vi "main.vi"() -> ()   [LabVIEW 2016]
uses:
  AlCS/Subsystems.ctl
  ts_labview_tcp/TCPClient/TCPClient.lvclass
  C:/Users/aanania/Documents/ts_alignmentsystemclient/ts_labview_tcp/TCPCommunicator/TCPCommunicator.lvclass
  ts_labview_tcp/TCPComEvents/TCPComEvents.lvclass
  ts_labview_tcp/TCPSettings/TCPSettings.lvclass
  AlCS/AlCS.lvclass
  ts_labview_tcp/tcpTypedefs/TCPSettings.ctl
  View/View.lvclass
  ts_labview_tcp/TCPComEvents/TCPComEvents.lvclass/TCPComEvents.ctl
  ts_labview_tcp/TCPCommunicator/TCPCommunicator.lvclass/TCPCommunicator.ctl
  AlCS/AlCS.lvclass/AlCS.ctl
  Parser/CommandCreator.lvclass
  ts_labview_tcp/TCPCommunicator/TCPCommunicator.lvclass
panel:
  out "connectedClicked":bool
  in  "stop":bool
  in  "SubsystemsPosition":T1
  in  "QueryPosition":bool
  in  "QueryLaserStatus":bool
  in  "PowerLaserOff":bool
  in  "ClearError":bool
  in  "QueryStatus":bool
  in  "execMP":bool
  in  "SubsystemsMP":T1
  out "String":string
  out "Connected":bool
  in  "Disconnect":bool
  in  "Connect":bool
  in  "timeout (ms)":i32=1500
  in  "port":u16=50000
  in  "IP":string="localhost"
  # "TCP Settings"
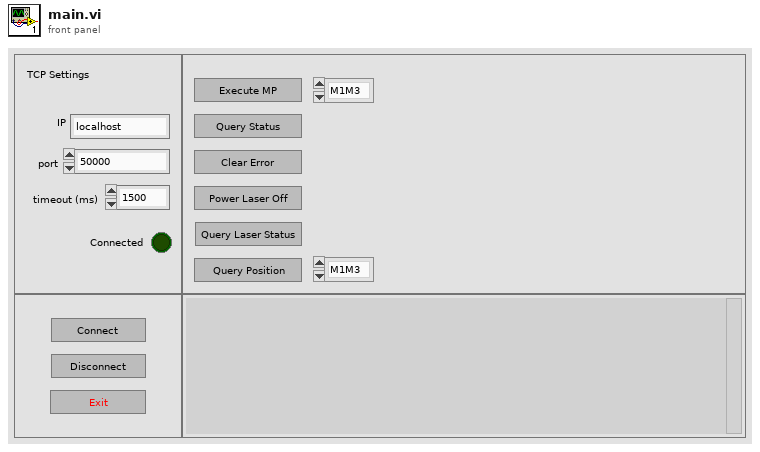
[diagram p1: front panel]
types:
  T1 = typedef "Subsystems.ctl" = enum16{"M1M3", "Camera", "M2"}
  T2 = typedef "TCPSettings.ctl" = cluster{"IP":string, "port_low":u16, "port_up":u16, "connection_timeout ":i32, "reading_timeout":i32, "writing_timeout":i32}
  T3 = cluster{"Subsystem":T1, "x":dbl, "y":dbl, "z":dbl, "rx":dbl, "ry":dbl, "rz":dbl}
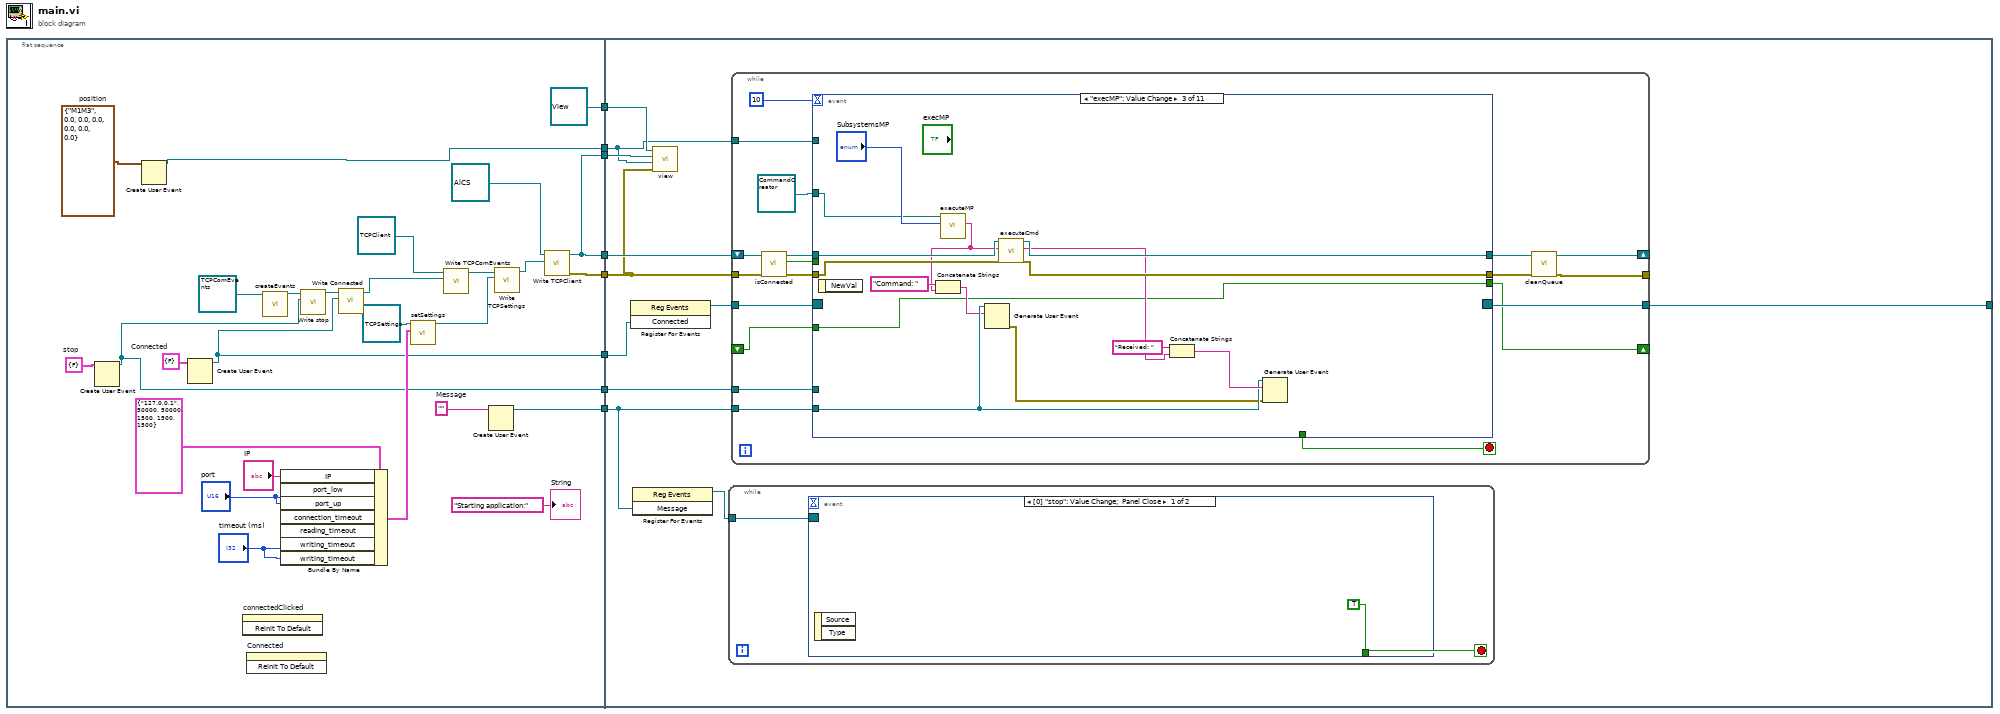
[diagram p0: block diagram]
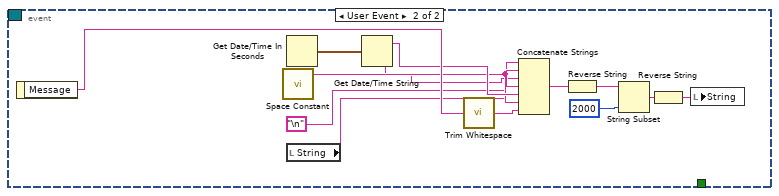
[diagram p2: hidden frame]
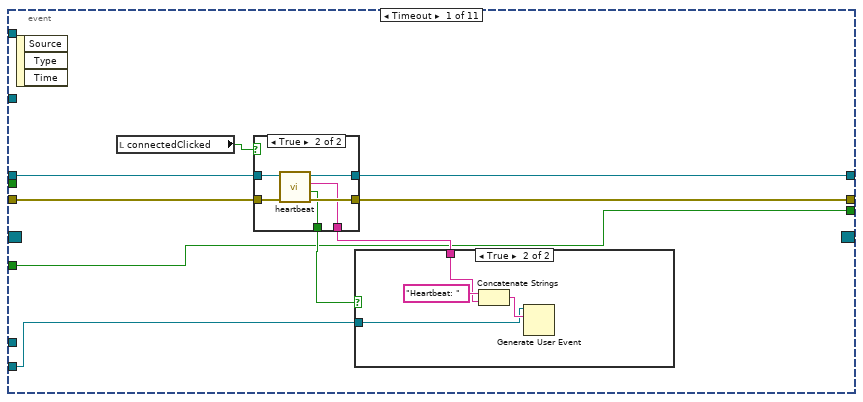
[diagram p3: hidden frame]
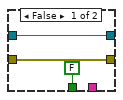
[diagram p5: hidden frame]
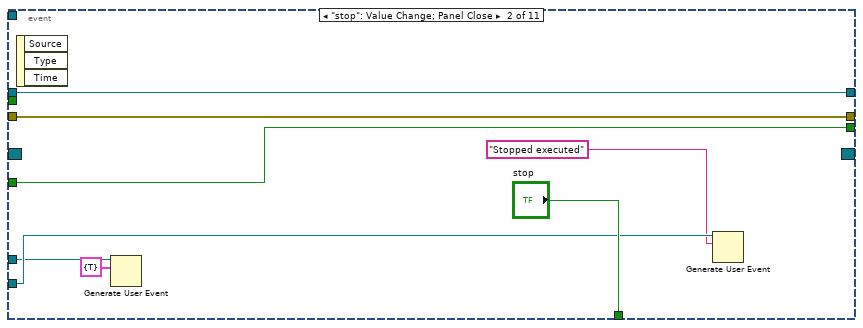
[diagram p6: hidden frame]
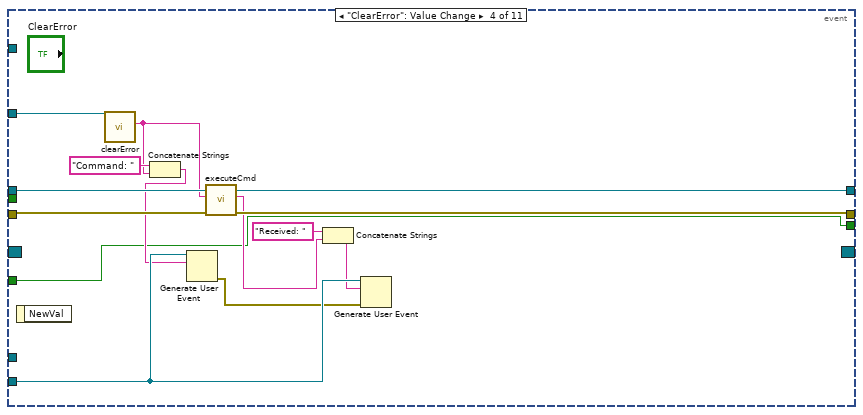
[diagram p7: hidden frame]
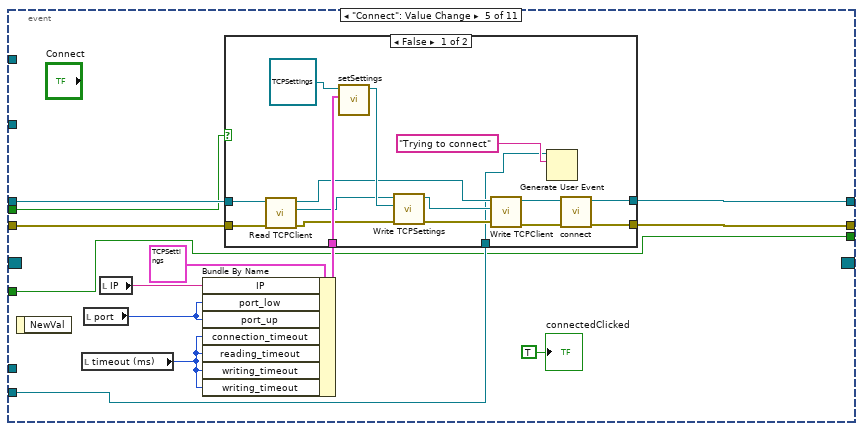
[diagram p8: hidden frame]
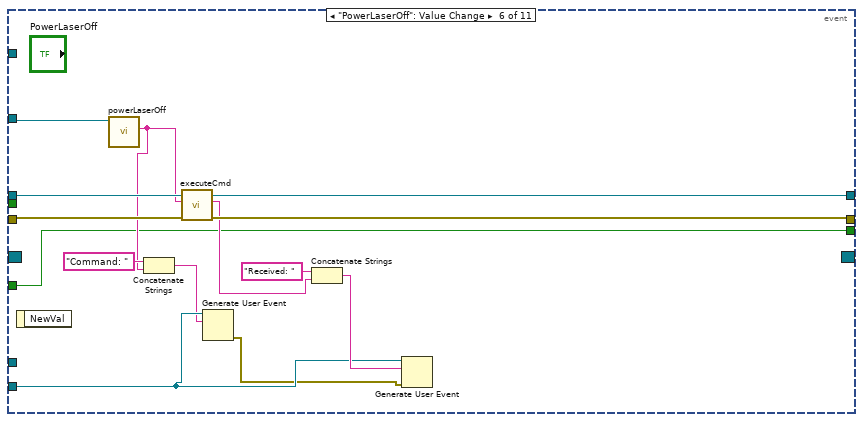
[diagram p10: hidden frame]
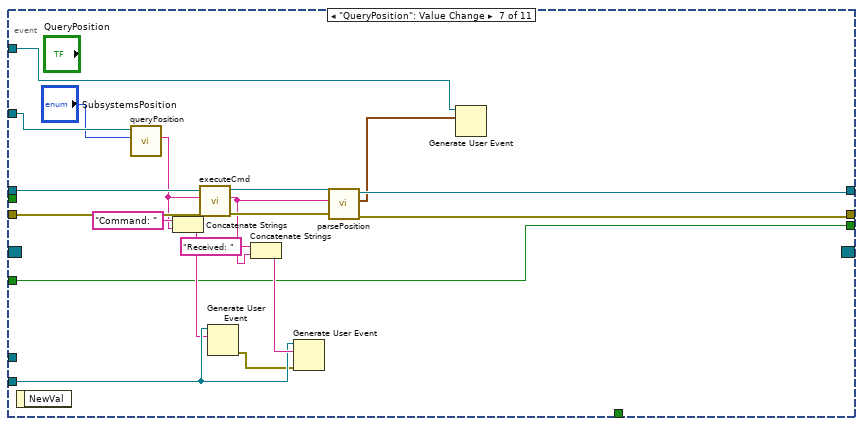
[diagram p11: hidden frame]
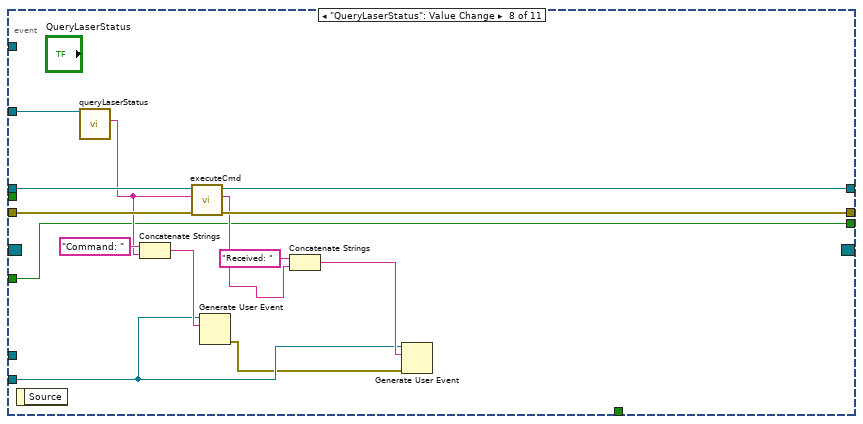
[diagram p12: hidden frame]
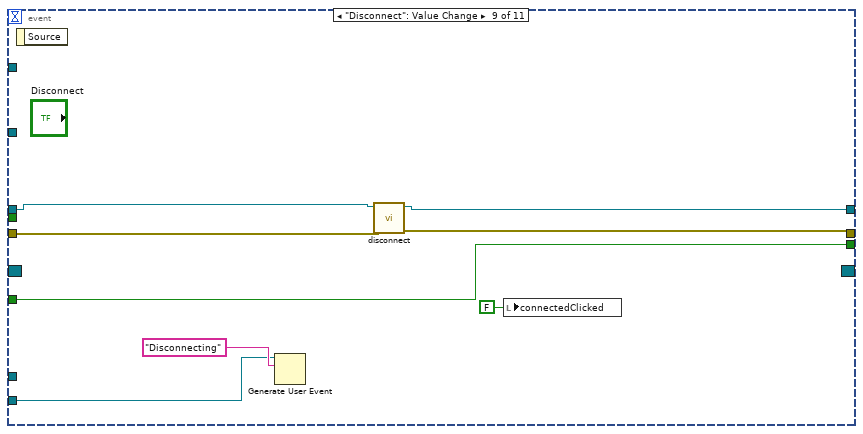
[diagram p13: hidden frame]
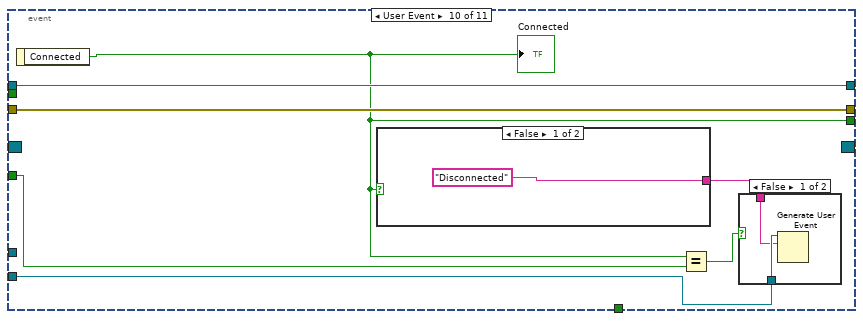
[diagram p14: hidden frame]
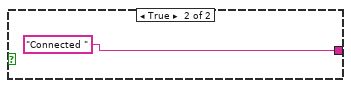
[diagram p16: hidden frame]
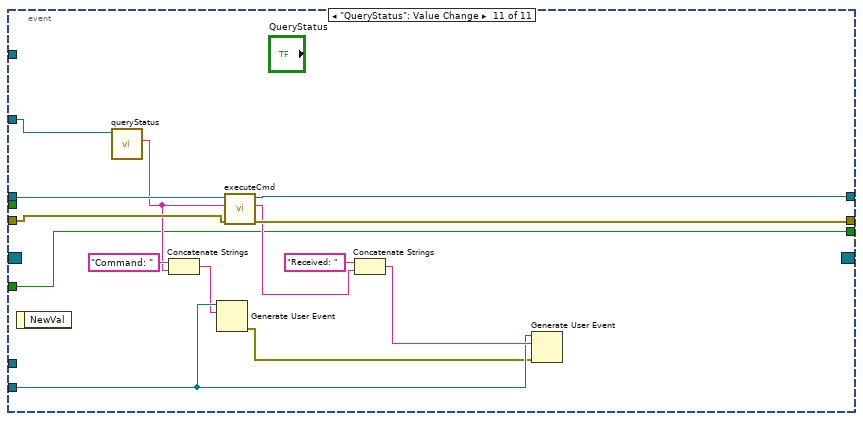
[diagram p17: hidden frame]
diagram:
  n1 = flat-sequence {
    tunnel: [w10] -> w8
    tunnel: [w19] -> w7
    tunnel: [w17] -> w6
    tunnel: [w16] -> w5
    tunnel: [w10] -> w4
    tunnel: [w12] -> w3
    tunnel: [refnum<class "View.lvclass"> refnum ("View in")] -> w2
    tunnel: [w9] -> w1
    tunnel: w8 -> [w43]
    tunnel: w7 -> [w46]
    tunnel: [w44] -> _
    tunnel: w6 -> [w39]
    tunnel: w5 -> [w41]
    tunnel: w4 -> [w40]
    tunnel: w3 -> [w36]
    tunnel: w2 -> [w38]
    tunnel: w1 -> [w37]
    frame #0 {
      w14 = T3 {"Subsystem"=enum."M1M3", "x"=0.0, "y"=0.0, "z"=0.0, "rx"=0.0, "ry"=0.0, "rz"=0.0}  # position
      w15 = ""  # Message
      w31 = cluster{"stop":bool} {"stop"=FALSE}  # stop
      w32 = cluster{"Connected":bool} {"Connected"=FALSE}  # Connected
      n2 = Create User Event(user event datatype=w31) -> (user event=w9:refnum<user-event>)  [unwired: 1 in, 1 out]
      n3 = Create User Event(user event datatype=w14) -> (user event=w12:refnum<user-event>)  [unwired: 1 in, 1 out]
      n4 = Create User Event(user event datatype=w32) -> (user event=w19:refnum<user-event>)  [unwired: 1 in, 1 out]
      n5 = invoke on="connectedClicked" class="Bool (strict)" method="Reinit To Default"() -> ()  [unwired: 3 in, 3 out]
      n6 = invoke on="Connected" class="Bool (strict)" method="Reinit To Default"() -> ()  [unwired: 3 in, 3 out]
      n7 = call "createEvents.vi"("TCPComEvents in"=refnum<class "TCPComEvents.lvclass"> refnum ("TCPComEvents.lvclass")) -> ("TCPComEvents out"=w30:refnum<class "TCPComEvents.lvclass">)  [unwired: 9 in, 1 out]
      n8 = Bundle By Name(cluster=T2 {"IP"="127.0.0.1", "port_low"=50000, "port_up"=50000, "connection_timeout "=1500, "reading_timeout"=1500, "writing_timeout"=1500} ("Cluster"), "IP"="IP", "port_low"="port", "port_up"="port", "connection_timeout"="timeout (ms)", "reading_timeout"="timeout (ms)", "writing_timeout"="timeout (ms)", "writing_timeout"="timeout (ms)") -> (w23:T2)
      n9 = call "Write stop.vi"("stop"=w9, "TCPComEvents in"=w30) -> ("TCPComEvents out"=w29:refnum<class "TCPComEvents.lvclass">)  [unwired: 8 in, 1 out]
      n10 = call "Write Connected.vi"("Connected"=w19, "TCPComEvents in"=w29) -> ("TCPComEvents out"=w28:refnum<class "TCPComEvents.lvclass">)  [unwired: 8 in, 1 out]
      n11 = call "setSettings.vi"("Settings"=w23, "TCPSettings in"=refnum<class "TCPSettings.lvclass"> refnum ("TCPSettings.lvclass")) -> ("TCPSettings out"=w26:refnum<class "TCPSettings.lvclass">)  [unwired: 8 in, 1 out]
      n12 = call "Write TCPComEvents.vi"("TCPComEvents.lvclass"=w28, "TCPCommunicator in"=refnum<class "TCPClient.lvclass"> refnum ("TCPClient.lvclass")) -> ("TCPCommunicator out"=w34:refnum<class "TCPClient.lvclass">)  [unwired: 8 in, 1 out]
      n13 = Create User Event(user event datatype=w15) -> (user event=w16:refnum<user-event>)  [unwired: 1 in, 1 out]
      n14 = call-dynamic "Write TCPSettings.vi"("TCPSettings.lvclass"=w26, "TCPCommunicator in"=w34) -> ("TCPCommunicator out"=w25:refnum<class "TCPClient.lvclass">)  [unwired: 8 in, 1 out]
      n15 = call "Write TCPClient.vi"("TCPClient.lvclass"=w25, "AlCS in"=refnum<class "AlCS.lvclass"> refnum ("AlCS.lvclass")) -> ("error out"=w17:errorcluster, "AlCS out"=w10:refnum<class "AlCS.lvclass">)  [unwired: 8 in]
      "String" <- "Starting application:" ("String")
    }
    frame #1 {
      n16 = register-events(w46) -> (reference out=w45:refnum<event-registration>)  [unwired: 2 in, 1 out]
      n17 = register-events(w41) -> (reference out=w42:refnum<event-registration>)  [unwired: 2 in, 1 out]
      n18 = call "view.vi"("error in (no error)"=w39, "positionEvent"=w36, "AlCS.lvclass"=w40, "View in"=w38) -> ()  [unwired: 6 in, 2 out]
      n19 = while {
        tunnel: w42 -> [w47]
        stop <- w48 stop-if-true
        n20 = event shown="[0] \"stop\": Value Change;  Panel Close" {
          selector: w47 -> [_ _]
          dyn-events: _ -> [_ _]
          timeout: _ -> [_ _]
          tunnel: [TRUE _] -> w48
          event "stop": Value Change; Panel Close {
            n21 = event-data() -> ()  [unwired: 1 in, 2 out]
          }
          event User Event {
            n22 = event-data() -> ("Message"=w62:string)  [unwired: 1 in]
            n23 = call <vilib>:"Space Constant.vi"() -> ("String"=w58:string)
            n24 = Get Date/Time In Seconds() -> (seconds since 1Jan1904=w60:timestamp)
            n25 = local read "String"() -> (w55:string)
            n26 = Get Date/Time String(seconds (now)=w60) -> (date string=w59:string, time string=w57:string)  [unwired: 2 in]
            n27 = call <vilib>:"Trim Whitespace.vi"("string"=w62) -> ("trimmed string"=w50:string)  [unwired: 1 in]
            n28 = Concatenate Strings(w55, "\n", w57, w58, w59, w58, w50) -> (w54:string)
            n29 = Reverse String(1:w54) -> (0:w53:string)
            n30 = String Subset(string=w53, length (rest)=2000 ("length (rest)")) -> (substring=w52:string)  [unwired: 1 in]
            n31 = Reverse String(1:w52) -> (0:w51:string)
            n32 = local write "String"(w51) -> ()
          }
        }
      }
      n33 = while {
        tunnel: w45 -> [w79]
        tunnel: [w78] -> w44
        tunnel: w39 -> [w73]
        shift-right: [w64] -> _
        shift-left: w43 -> [w77]
        shift-right: [w69] -> _
        shift-left: _ -> [w71]
        tunnel: w41 -> [w70]
        tunnel: w37 -> [w68]
        tunnel: w36 -> [w67]
        tunnel: [w63] -> _
        stop <- w80 stop-if-true
        n34 = call "isConnected.vi"("error in (no error)"=w73, "AlCS in"=w77) -> ("error out"=w74:errorcluster, "conneced?"=w75:bool, "AlCS out"=w76:refnum<class "AlCS.lvclass">)  [unwired: 7 in]
        n35 = event shown="[2] \"execMP\": Value Change" {
          selector: w79 -> [_ _ _ _ _ _ _ _ _ _ _]
          dyn-events: [_ _ _ _ _ _ _ _ _ _ _] -> w78
          timeout: 10 -> [_ _ _ _ _ _ _ _ _ _ _]
          tunnel: [_ "stop" _ _ _ _ _ _ _ _ _] -> w80
          tunnel: w76 -> [w90 w110 w124 w139 w146 w184 w202 w217 w224 w233 w250]
          tunnel: w75 -> [_ _ _ _ w144 _ _ _ _ _ _]
          tunnel: w74 -> [w89 w109 w123 w138 w145 w183 w201 w216 w223 w232 w249]
          tunnel: [w88 w109 w122 w137 w153 w182 w188 w215 w226 w232 w248] -> w66
          tunnel: [w87 w110 w121 w136 w152 w181 w189 w214 w225 w233 w247] -> w65
          tunnel: refnum<class "CommandCreator.lvclass"> refnum ("CommandCreator.lvclass") -> [_ _ w125 w140 _ w185 w204 w218 _ _ w251]
          tunnel: w71 -> [w82 w106 w112 w127 w141 w172 w193 w205 w219 w231 w238]
          tunnel: w70 -> [w85 w108 w115 w133 w142 w175 w196 w207 w220 w229 w241]
          tunnel: [w82 w106 w112 w127 w141 w172 w193 w205 w219 w227 w238] -> w69
          tunnel: w68 -> [_ w105 _ _ _ _ _ _ _ _ _]
          tunnel: w67 -> [_ _ _ _ _ _ w187 _ _ _ _]
          event Timeout {
            n36 = event-data() -> ()  [unwired: 1 in, 3 out]
            n37 = local read "connectedClicked"() -> (w86:bool)
            n38 = case shown="True" w86 {
              tunnel: w90 -> [w97 w103]
              tunnel: w89 -> [w96 w102]
              tunnel: [w96 w101] -> w88
              tunnel: [w97 w100] -> w87
              tunnel: [_ w99] -> w84
              tunnel: [FALSE ("newValue") w98] -> w83
              frame False {
              }
              frame True {
                n39 = call "heartbeat.vi"("error in (no error)"=w102, "AlCS in"=w103) -> ("error out"=w101:errorcluster, "newValue"=w98:bool, "answer"=w99:string, "AlCS out"=w100:refnum<class "AlCS.lvclass">)  [unwired: 6 in]
              }
            }
            n40 = case shown="True" w83 {
              tunnel: w85 -> [_ w92]
              tunnel: w84 -> [_ w91]
              frame False {
              }
              frame True {
                n41 = Concatenate Strings("Heartbeat: " ("string"), w91) -> (w93:string)
                n42 = Generate User Event(user event=w92, event data cluster=w93) -> ()  [unwired: 2 in, 2 out]
              }
            }
          }
          event "stop": Value Change; Panel Close {
            n43 = event-data() -> ()  [unwired: 1 in, 3 out]
            n44 = Generate User Event(user event=w105, event data cluster=cluster{"stop":bool} {"stop"=TRUE} ("event data")) -> ()  [unwired: 2 in, 2 out]
            n45 = Generate User Event(user event=w108, event data cluster="Stopped executed" ("answer")) -> ()  [unwired: 2 in, 2 out]
          }
          event "execMP": Value Change {
            n46 = event-data() -> ()  [unwired: 1 in, 1 out]
            n47 = call "executeMP.vi"("Subsystems"="SubsystemsMP", "Parser in"=w125) -> ("command"=w116:string)  [unwired: 7 in, 2 out]
            n48 = Concatenate Strings("Command: " ("string"), w116) -> (w114:string)
            n49 = Generate User Event(user event=w115, event data cluster=w114) -> (error out=w113:errorcluster)  [unwired: 2 in, 1 out]
            n50 = call "executeCmd.vi"("error in (no error)"=w123, "command"=w116, "AlCS in"=w124) -> ("error out"=w122:errorcluster, "answer"=w119:string, "AlCS out"=w121:refnum<class "AlCS.lvclass">)  [unwired: 6 in]
            n51 = Concatenate Strings("Received: " ("string"), w119) -> (w118:string)
            n52 = Generate User Event(user event=w115, event data cluster=w118, error in=w113) -> ()  [unwired: 1 in, 2 out]
          }
          event "ClearError": Value Change {
            n53 = event-data() -> ()  [unwired: 1 in, 1 out]
            n54 = call "clearError.vi"("CommandCreator in"=w140) -> ("command"=w134:string)  [unwired: 8 in, 2 out]
            n55 = Concatenate Strings("Command: " ("string"), w134) -> (w132:string)
            n56 = Generate User Event(user event=w133, event data cluster=w132) -> (error out=w128:errorcluster)  [unwired: 2 in, 1 out]
            n57 = call "executeCmd.vi"("error in (no error)"=w138, "command"=w134, "AlCS in"=w139) -> ("error out"=w137:errorcluster, "answer"=w130:string, "AlCS out"=w136:refnum<class "AlCS.lvclass">)  [unwired: 6 in]
            n58 = Concatenate Strings("Received: " ("string"), w130) -> (w129:string)
            n59 = Generate User Event(user event=w133, event data cluster=w129, error in=w128) -> ()  [unwired: 1 in, 2 out]
          }
          event "Connect": Value Change {
            n60 = event-data() -> ()  [unwired: 1 in, 1 out]
            n61 = local read "timeout (ms)"() -> (w148:i32)
            n62 = local read "port"() -> (w149:u16)
            n63 = local read "IP"() -> (w150:string)
            n64 = Bundle By Name(cluster=T2 {"IP"="127.0.0.1", "port_low"=50000, "port_up"=50000, "connection_timeout "=1500, "reading_timeout"=1500, "writing_timeout"=1500} ("Cluster"), "IP"=w150, "port_low"=w149, "port_up"=w149, "connection_timeout"=w148, "reading_timeout"=w148, "writing_timeout"=w148, "writing_timeout"=w148) -> (w147:T2)
            n65 = case shown="False" w144 {
              tunnel: [w169 w170] -> w153
              tunnel: [w168 w171] -> w152
              tunnel: w147 -> [w166 _]
              tunnel: w146 -> [w164 w171]
              tunnel: w145 -> [w163 w170]
              tunnel: w142 -> [w154 _]
              frame False {
                n66 = call "Read TCPClient.vi"("error in (no error)"=w163, "AlCS in"=w164) -> ("error out"=w160:errorcluster, "TCPClient.lvclass"=w161:refnum<class "TCPClient.lvclass">, "AlCS out"=w162:refnum<class "AlCS.lvclass">)  [unwired: 7 in]
                n67 = call "setSettings.vi"("Settings"=w166, "TCPSettings in"=refnum<class "TCPSettings.lvclass"> refnum ("TCPSettings.lvclass")) -> ("TCPSettings out"=w165:refnum<class "TCPSettings.lvclass">)  [unwired: 8 in, 1 out]
                n68 = call-dynamic "Write TCPSettings.vi"("error in (no error)"=w160, "TCPSettings.lvclass"=w165, "TCPCommunicator in"=w161) -> ("error out"=w159:errorcluster, "TCPCommunicator out"=w158:refnum<class "TCPClient.lvclass">)  [unwired: 7 in]
                n69 = call "Write TCPClient.vi"("error in (no error)"=w159, "TCPClient.lvclass"=w158, "AlCS in"=w162) -> ("error out"=w157:errorcluster, "AlCS out"=w156:refnum<class "AlCS.lvclass">)  [unwired: 7 in]
                n70 = Generate User Event(user event=w154, event data cluster="Trying to connect" ("answer")) -> ()  [unwired: 2 in, 2 out]
                n71 = call "connect.vi"("error in (no error)"=w157, "AlCS in"=w156) -> ("error out"=w169:errorcluster, "AlCS out"=w168:refnum<class "AlCS.lvclass">)  [unwired: 8 in]
              }
              frame True {
              }
            }
            "connectedClicked" <- TRUE ("connectedClicked")
          }
          event "PowerLaserOff": Value Change {
            n72 = event-data() -> ()  [unwired: 1 in, 1 out]
            n73 = call "powerLaserOff.vi"("Parser in"=w185) -> ("command"=w176:string)  [unwired: 8 in, 2 out]
            n74 = Concatenate Strings("Command: " ("string"), w176) -> (w174:string)
            n75 = call "executeCmd.vi"("error in (no error)"=w183, "command"=w176, "AlCS in"=w184) -> ("error out"=w182:errorcluster, "answer"=w179:string, "AlCS out"=w181:refnum<class "AlCS.lvclass">)  [unwired: 6 in]
            n76 = Generate User Event(user event=w175, event data cluster=w174) -> (error out=w173:errorcluster)  [unwired: 2 in, 1 out]
            n77 = Concatenate Strings("Received: " ("string"), w179) -> (w178:string)
            n78 = Generate User Event(user event=w175, event data cluster=w178, error in=w173) -> ()  [unwired: 1 in, 2 out]
          }
          event "QueryPosition": Value Change {
            n79 = event-data() -> ()  [unwired: 1 in, 1 out]
            n80 = call "queryPosition.vi"("Subsystems"="SubsystemsPosition", "CommandCreator in"=w204) -> ("command"=w197:string)  [unwired: 7 in, 2 out]
            n81 = Concatenate Strings("Command: " ("string"), w197) -> (w195:string)
            n82 = call "executeCmd.vi"("error in (no error)"=w201, "command"=w197, "AlCS in"=w202) -> ("error out"=w192:errorcluster, "answer"=w191:string, "AlCS out"=w190:refnum<class "AlCS.lvclass">)  [unwired: 6 in]
            n83 = Generate User Event(user event=w196, event data cluster=w195) -> (error out=w194:errorcluster)  [unwired: 2 in, 1 out]
            n84 = Concatenate Strings("Received: " ("string"), w191) -> (w199:string)
            n85 = Generate User Event(user event=w196, event data cluster=w199, error in=w194) -> ()  [unwired: 1 in, 2 out]
            n86 = call "parsePosition.vi"("error in (no error)"=w192, "position"=w191, "AlCS in"=w190) -> ("error out"=w188:errorcluster, "position"=w186:T3, "AlCS out"=w189:refnum<class "AlCS.lvclass">)  [unwired: 6 in]
            n87 = Generate User Event(user event=w187, event data cluster=w186) -> ()  [unwired: 2 in, 2 out]
          }
          event "QueryLaserStatus": Value Change {
            n88 = event-data() -> ()  [unwired: 1 in, 1 out]
            n89 = call "queryLaserStatus.vi"("CommandCreator in"=w218) -> ("command"=w209:string)  [unwired: 8 in, 2 out]
            n90 = Concatenate Strings("Command: " ("string"), w209) -> (w208:string)
            n91 = call "executeCmd.vi"("error in (no error)"=w216, "command"=w209, "AlCS in"=w217) -> ("error out"=w215:errorcluster, "answer"=w212:string, "AlCS out"=w214:refnum<class "AlCS.lvclass">)  [unwired: 6 in]
            n92 = Generate User Event(user event=w207, event data cluster=w208) -> (error out=w206:errorcluster)  [unwired: 2 in, 1 out]
            n93 = Concatenate Strings("Received: " ("string"), w212) -> (w211:string)
            n94 = Generate User Event(user event=w207, event data cluster=w211, error in=w206) -> ()  [unwired: 1 in, 2 out]
          }
          event "Disconnect": Value Change {
            n95 = event-data() -> ()  [unwired: 1 in, 1 out]
            n96 = Generate User Event(user event=w220, event data cluster="Disconnecting" ("answer")) -> ()  [unwired: 2 in, 2 out]
            n97 = call "disconnect.vi"("error in (no error)"=w223, "AlCS in"=w224) -> ("error out"=w226:errorcluster, "AlCS out"=w225:refnum<class "AlCS.lvclass">)  [unwired: 8 in]
            n98 = local write "connectedClicked"(FALSE ("connectedClicked")) -> ()
          }
          event User Event {
            n99 = event-data() -> ("Connected"=w227:bool)  [unwired: 1 in]
            "Connected" <- w227
            n100 = case shown="False" w227 {
              tunnel: ["Disconnected" ("answer") "Connected " ("answer")] -> w228
              frame False {
              }
              frame True {
              }
            }
            n101 = Equal?(x=w227, y=w231) -> (x = y?=w230:bool)
            n102 = case shown="False" w230 {
              tunnel: w229 -> [w235 _]
              tunnel: w228 -> [w234 _]
              frame False {
                n103 = Generate User Event(user event=w235, event data cluster=w234) -> ()  [unwired: 2 in, 2 out]
              }
              frame True {
              }
            }
          }
          event "QueryStatus": Value Change {
            n104 = event-data() -> ()  [unwired: 1 in, 1 out]
            n105 = call "queryStatus.vi"("CommandCreator in"=w251) -> ("command"=w242:string)  [unwired: 8 in, 2 out]
            n106 = Concatenate Strings("Command: " ("string"), w242) -> (w240:string)
            n107 = Generate User Event(user event=w241, event data cluster=w240) -> (error out=w239:errorcluster)  [unwired: 2 in, 1 out]
            n108 = call "executeCmd.vi"("error in (no error)"=w249, "command"=w242, "AlCS in"=w250) -> ("error out"=w248:errorcluster, "answer"=w245:string, "AlCS out"=w247:refnum<class "AlCS.lvclass">)  [unwired: 6 in]
            n109 = Concatenate Strings("Received: " ("string"), w245) -> (w244:string)
            n110 = Generate User Event(user event=w241, event data cluster=w244, error in=w239) -> ()  [unwired: 1 in, 2 out]
          }
        }
        n111 = call "cleanQueue.vi"("error in (no error)"=w66, "AlCS in"=w65) -> ("error out"=w63:errorcluster, "AlCS out"=w64:refnum<class "AlCS.lvclass">)  [unwired: 7 in, 1 out]
      }
    }
  }
